vi "ziLoadFactory.vi"(4 "error in":errorcluster, 7 "Handle In":T1 {"Handle" format="0x%08x"; "Conn" format="0x%08x"}) -> (0 "error out":errorcluster, 3 "Handle Out":T1 {"Handle" format="0x%08x"; "Conn" format="0x%08x"})   [LabVIEW 2009, in "Zurich Instruments LabOne.lvlib"]
doc: "This resets the device to factory default. Warning: HF2 not supported"
uses:
  <instrlib>/Zurich Instruments LabOne/Zurich Instruments LabOne.lvlib
  <instrlib>/Zurich Instruments LabOne/Public/ziTypeHandle.ctl
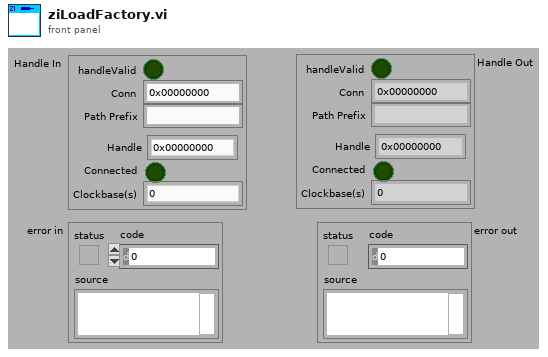
[diagram p1: front panel]
types:
  T1 = typedef "Zurich Instruments LabOne.lvlib/ziTypeHandle.ctl" = cluster{"handleValid":bool, "Conn":u64, "Path Prefix":string, "Handle":u64, "Connected":bool, "Clockbase(s)":dbl}
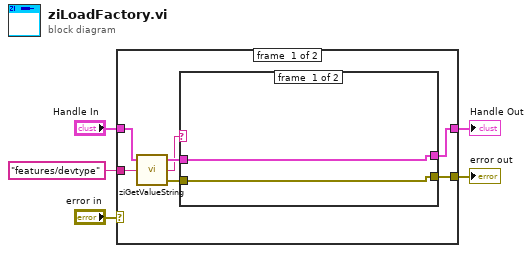
[diagram p0: block diagram]
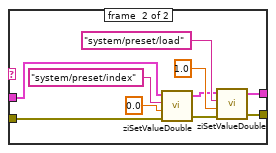
[diagram p2: hidden frame]
diagram:
  n1 = case shown="Error" "error in" {
    selector: "error in" -> [_ w25]
    tunnel: [w12 w25] -> w5
    tunnel: [w11 w26] -> w4
    tunnel: "features/devtype" ("Path") -> [w10 _]
    tunnel: "Handle In" -> [w8 w26]
    frame #0 {
      n2 = call <instrlib>:"ziGetValueString.vi"("Path"=w10, "Handle In"=w8) -> ("error out"=w9:errorcluster, "Value"=w6:string, "Handle Out"=w7:T1)  [unwired: 1 in]
      n3 = case shown="\"HF2LI\"" w6 {
        tunnel: [w13 w23] -> w12
        tunnel: [w14 w17] -> w11
        tunnel: w9 -> [w13 w16]
        tunnel: w7 -> [w14 w15]
        frame #0 {
        }
        frame #1 {
          n4 = call <instrlib>:"ziSetValueDouble.vi"("Error In"=w16, "Value"=0.0, "Path"="system/preset/index", "Handle In"=w15) -> ("Error Out"=w24:errorcluster, "Handle Out"=w18:T1)  [unwired: 1 in]
          n5 = call <instrlib>:"ziSetValueDouble.vi"("Error In"=w24, "Value"=1.0, "Path"="system/preset/load", "Handle In"=w18) -> ("Error Out"=w23:errorcluster, "Handle Out"=w17:T1)  [unwired: 1 in]
        }
      }
    }
    frame #1 {
    }
  }
  "Handle Out" <- w4
  "error out" <- w5
